vi "Configure Power Signals.vi"(0 "VISA resource name":refnum<visa-resource-name>, 1 "Overshoot Voltage (5 Percent)":i32=5, 2 "Expected Steady Voltage (20 V)":dbl=20.0, 5 "Cycles Number (1)":i32=1, 7 "Duration Time (1E-6 Second)":dbl=1e-06, 9 "Expected Inrush Current (2 A)":dbl=2.0, 11 "error in (no error)":errorcluster, 12 "Expected Maximum Voltage (20 V)":dbl=20.0) -> (4 "VISA resource name out":refnum<visa-resource-name>, 15 "error out":errorcluster)   [LabVIEW 2016, in "Agilent 2000 3000 X-Series.lvlib"]
doc: "Configure the Power Signals settings."
uses:
  Agilent 2000 3000 X-Series.lvlib
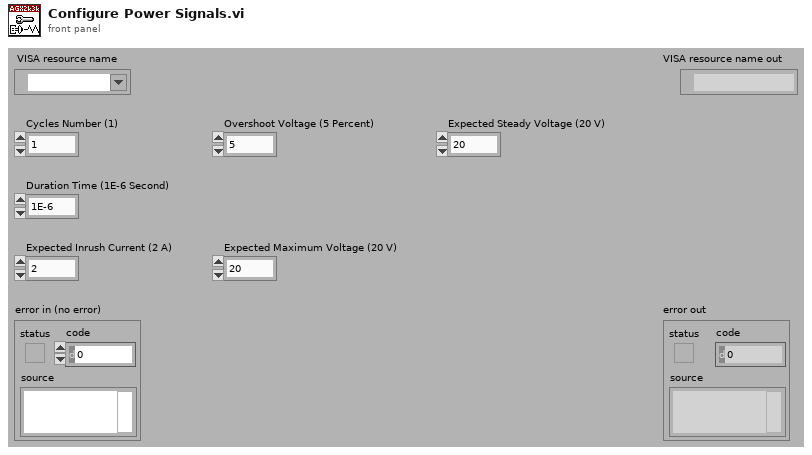
[diagram p1: front panel]
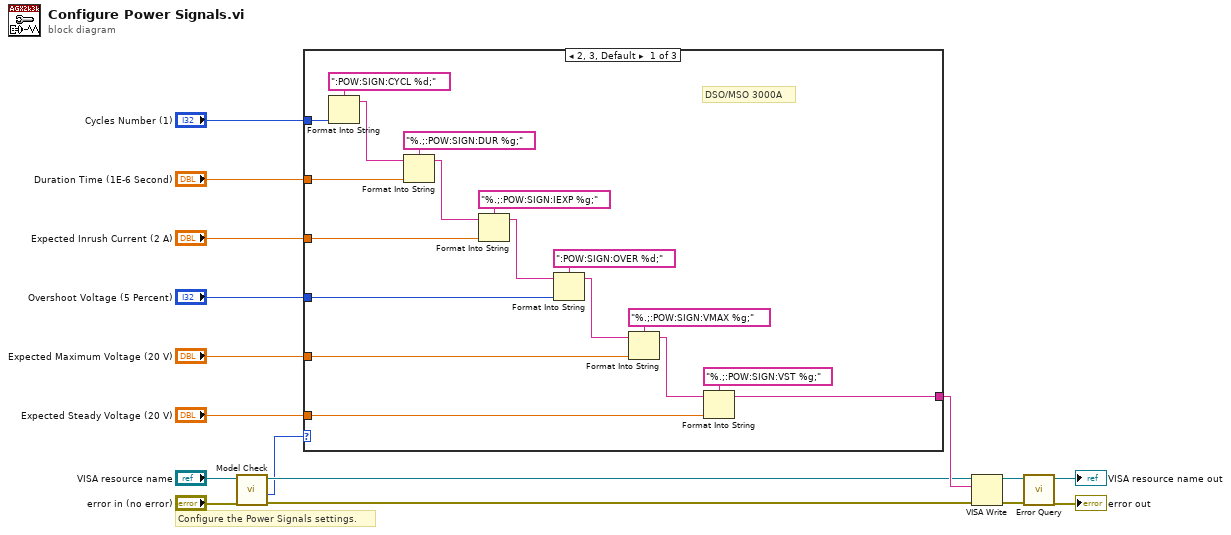
[diagram p0: block diagram]
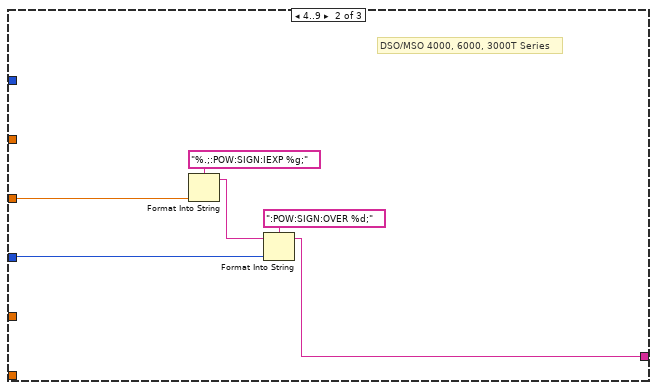
[diagram p2: hidden frame]
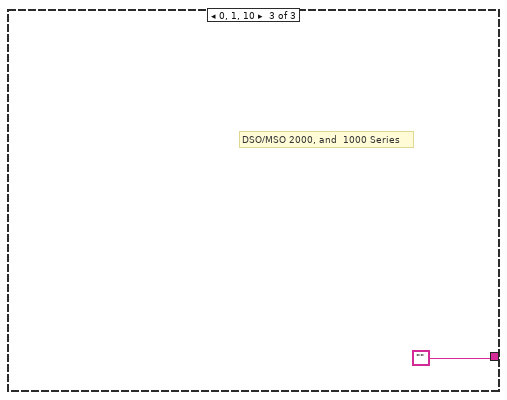
[diagram p3: hidden frame]
diagram:
  # "Configure the Power Signals settings."
  n1 = call "Model Check.vi"("error in (no error)"="error in (no error)", "VISA resource name"="VISA resource name") -> ("error out"=w2:errorcluster, "Model"=w1:i32, "VISA resource name out"=w3:refnum<visa-resource-name>)  [unwired: 7 out]
  n2 = case shown="2, 3, Default" w1 {
    tunnel: "Cycles Number (1)" -> [w24 _ _]
    tunnel: "Duration Time (1E-6 Second)" -> [w23 _ _]
    tunnel: "Expected Inrush Current (2 A)" -> [w22 w37 _]
    tunnel: "Overshoot Voltage (5 Percent)" -> [w20 w36 _]
    tunnel: "Expected Maximum Voltage (20 V)" -> [w19 _ _]
    tunnel: "Expected Steady Voltage (20 V)" -> [w18 _ _]
    tunnel: [w17 w35 ""] -> w4
    frame 2, 3, Default {
      # "DSO/MSO 3000A"
      n3 = Format Into String(format string=":POW:SIGN:CYCL %d;", w24) -> (resulting string=w34:string)  [unwired: 2 in, 1 out]
      n4 = Format Into String(format string="%.;:POW:SIGN:DUR %g;", initial string=w34, w23) -> (resulting string=w32:string)  [unwired: 1 in, 1 out]
      n5 = Format Into String(format string="%.;:POW:SIGN:IEXP %g;", initial string=w32, w22) -> (resulting string=w30:string)  [unwired: 1 in, 1 out]
      n6 = Format Into String(format string=":POW:SIGN:OVER %d;", initial string=w30, w20) -> (resulting string=w28:string)  [unwired: 1 in, 1 out]
      n7 = Format Into String(format string="%.;:POW:SIGN:VMAX %g;", initial string=w28, w19) -> (resulting string=w26:string)  [unwired: 1 in, 1 out]
      n8 = Format Into String(format string="%.;:POW:SIGN:VST %g;", initial string=w26, w18) -> (resulting string=w17:string)  [unwired: 1 in, 1 out]
    }
    frame 4..9 {
      # "DSO/MSO 4000, 6000, 3000T Series"
      n9 = Format Into String(format string="%.;:POW:SIGN:IEXP %g;", w37) -> (resulting string=w39:string)  [unwired: 2 in, 1 out]
      n10 = Format Into String(format string=":POW:SIGN:OVER %d;", initial string=w39, w36) -> (resulting string=w35:string)  [unwired: 1 in, 1 out]
    }
    frame 0, 1, 10 {
      # "DSO/MSO 2000, and  1000 Series"
    }
  }
  n11 = VISA Write(VISA resource name=w3, write buffer=w4, error in (no error)=w2) -> (VISA resource name out=w16:refnum<visa-resource-name>, error out=w15:errorcluster)  [unwired: 1 out]
  n12 = call "Error Query.vi"("error in (no error)"=w15, "VISA resource name"=w16) -> ("error out"=→"error out":errorcluster, "VISA resource name out"=→"VISA resource name out":refnum<visa-resource-name>)  [unwired: 8 out]
